vi "check should pass.vi"() -> ()   [LabVIEW 2016]
uses:
  Source/JSON Value/JSON Value.lvclass
panel:
  out "Failed results (there should be none, all should be passes)":T1(array[cluster])
  out "All Results":T1(array[cluster])
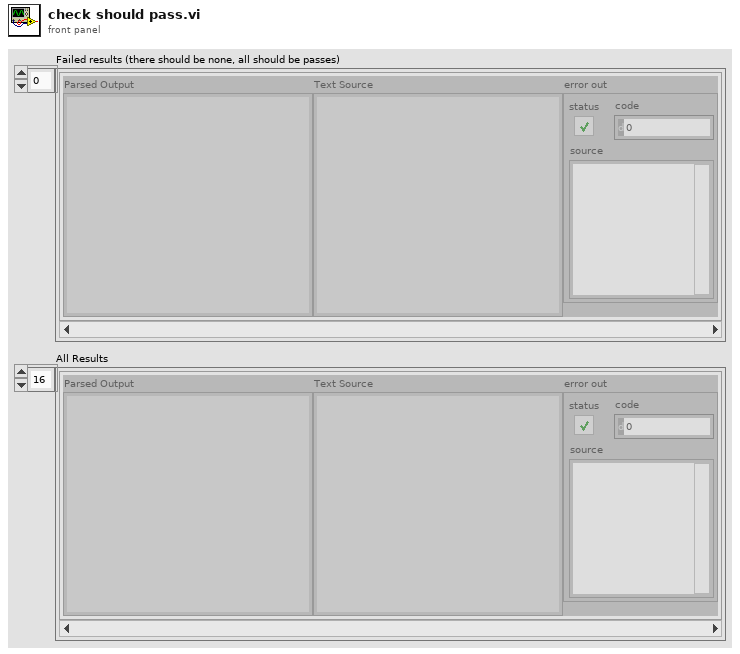
[diagram p1: front panel]
types:
  T1 = cluster{"Parsed Output":string, "Text Source":string, "error out":errorcluster}[]
  T2 = cluster{"String":string, string, "error out":errorcluster}
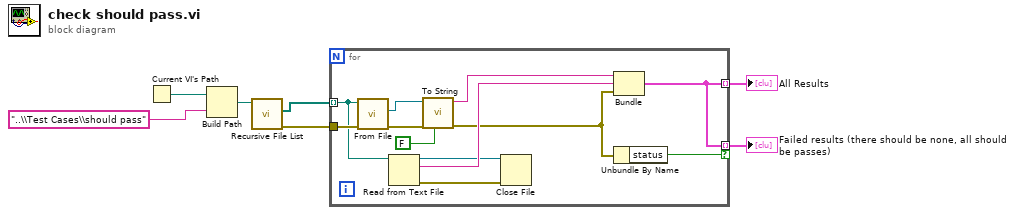
[diagram p0: block diagram]
diagram:
  n1 = Current VI's Path() -> (path=w1:path)
  n2 = Build Path(base path=w1, name or relative path="..\\Test Cases\\should pass" ("Path")) -> (appended path=w2:path)
  n3 = call <vilib>:"Recursive File List.vi"("Folder Path"=w2) -> ("error out"=w6:errorcluster, "All Files in Dir"=w4:path[])  [unwired: 6 in, 3 out]
  n4 = for {
    tunnel: w4 -> [w16] mode=indexing
    tunnel: w6 -> [w18]
    tunnel: [w12] -> w5 mode=indexing
    tunnel: [w12] -> w3 mode=indexing if=w10
    n5 = call "From File.vi"("error in"=w18, "file path"=w16) -> ("error out"=w17:errorcluster, "JSON Value out"=w19:refnum<class "JSON Value.lvclass">)  [unwired: 8 in]
    n6 = Read from Text File(file (use dialog)=w16) -> (refnum out=w9:refnum<file>, text=w14:string, error out=w8:errorcluster)  [unwired: 3 in, 1 out]
    n7 = call "To String.vi"("pretty print? (F)"=FALSE ("pretty print? (T)"), "error in (no error)"=w17, "JSON Value in"=w19) -> ("error out"=w11:errorcluster, "String"=w15:string)  [unwired: 7 in]
    n8 = Close File(refnum=w9, error in=w8) -> ()  [unwired: 2 out]
    n9 = Bundle("String"=w15, w14, "error out"=w11) -> (w12:T2)  [unwired: 1 in]
    n10 = Unbundle By Name(w11) -> ("status"=w10:bool)
  }
  "All Results" <- w5
  "Failed results (there should be none, all should be passes)" <- w3
